vi "Read SCL Transition.vi"(8 "error in (no error)":errorcluster, 11 "TX Speed in":refnum<class "TX Speed.lvclass">) -> (0 "error out":errorcluster, 2 "SCL Transition":u32[](array[numeric]), 3 "TX Speed out":refnum<class "TX Speed.lvclass">)   [LabVIEW 2020, in "TX Speed.lvclass"]
uses:
  TX Speed.lvclass
  TX Speed.lvclass/TX Speed.ctl
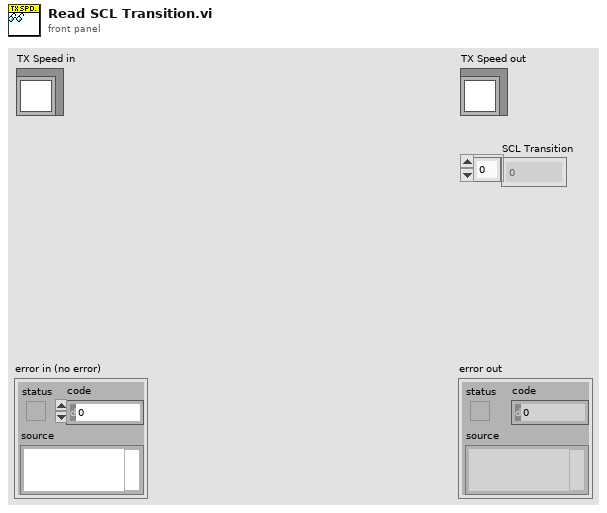
[diagram p1: front panel]
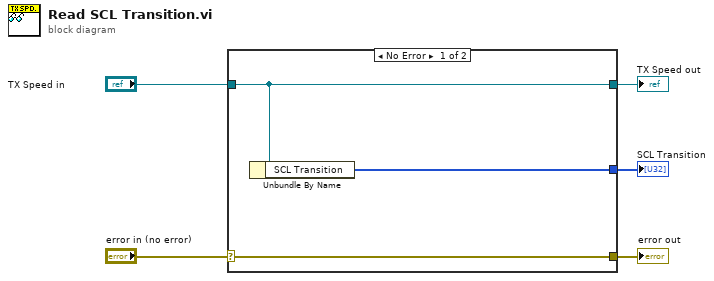
[diagram p0: block diagram]
diagram:
  n1 = case shown="No Error" "error in (no error)" {
    selector: "error in (no error)" -> [w8 w9]
    tunnel: [w8 w9] -> w4
    tunnel: [w7 w10] -> w2
    tunnel: "TX Speed in" -> [w7 w10]
    tunnel: [w6 _] -> w1
    frame No Error {
      n2 = Unbundle By Name(w7) -> ("SCL Transition"=w6:u32[])
    }
    frame Error {
    }
  }
  "error out" <- w4
  "TX Speed out" <- w2
  "SCL Transition" <- w1
